vi "DHE_set_pixtime.vi"(0 "fd":i32, 7 "time":sgl, 11 "error in (no error)":errorcluster) -> (4 "fd out":i32, 8 "return value":i32, 15 "error out":errorcluster)   [LabVIEW 2016]
doc: "This VI turns instrument power on (Flag=1) or off (Flag=0)."
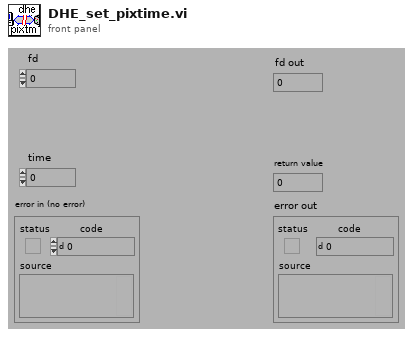
[diagram p1: front panel]
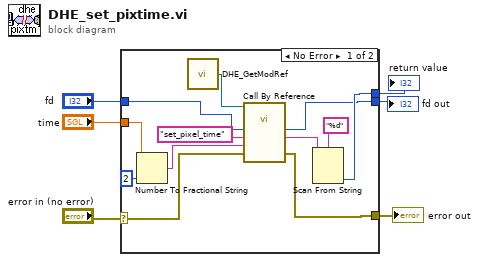
[diagram p0: block diagram]
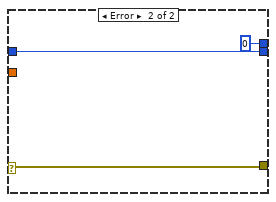
[diagram p2: hidden frame]
diagram:
  n1 = case shown="No Error" "error in (no error)" {
    selector: "error in (no error)" -> [w13 w19]
    tunnel: "fd" -> [w14 w21]
    tunnel: [w11 0] -> w5
    tunnel: [w12 w19] -> w4
    tunnel: "time" -> [w9 _]
    tunnel: [w10 w21] -> w2
    frame No Error {
      n2 = Number To Fractional String(number=w9, precision (6)=i16 2) -> (F-format string=w8:string)  [unwired: 2 out]
      n3 = call "DHE_GetModRef.vi"() -> ("DHE_ModRef"=w18:refnum<vi>)  [unwired: 9 out]
      n4 = call-by-ref "?"(reference=w18, "error in (no error)"=w13, "arguments"=w8, "function"="set_pixel_time", "fd in"=w14) -> ("error out"=w12:errorcluster, "str result"=w16:string, "fd out"=w10:i32)  [unwired: 5 in, 3 out]
      n5 = Scan From String(format string="%d", input string=w16) -> (output 1=w11:i32)  [unwired: 2 in, 4 out]
    }
    frame Error {
    }
  }
  "error out" <- w4
  "return value" <- w5
  "fd out" <- w2
